vi "Configuration - Read All Module Configurations of a Specific Type.vi"(8 "error in":errorcluster, 10 "Module Type":T2=enum."Analog In Module") -> (0 "error out":errorcluster, 2 "Module Configurations":T1[](array[typedef]), 3 "Carrier Control Port":i32)   [LabVIEW 2017, in "Communications Library.lvlib"]
uses:
  Communications Library.lvlib
  Typedefs/DTACQ Device Type--Enum.ctl
  Typedefs/DTACQ Module Configuration--Cluster.ctl
  Typedefs/Functional Global Variable Action--Enum.ctl
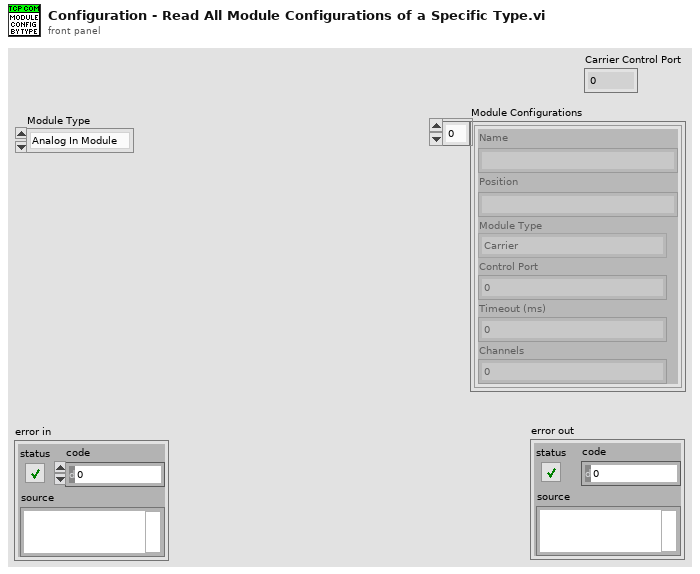
[diagram p1: front panel]
types:
  T1 = typedef "Communications Library.lvlib/DTACQ Module Configuration--Cluster.ctl" = cluster{"Name":string, "Position":string, "Module Type":T2, "Control Port":i32, "Timeout (ms)":i32, "Channels":i32}
  T2 = typedef "Communications Library.lvlib/DTACQ Device Type--Enum.ctl" = enum16{"Carrier", "Analog In Module", "Analog Out Module", "Generic Module"}
  T3 = typedef "Communications Library.lvlib/Functional Global Variable Action--Enum.ctl" = enum16{"Initialise", "Write Module Config", "Write Carrier Config", "Read"}
  T4 = typedef "Communications Library.lvlib/DTACQ Module Carrier Configuration--Cluster.ctl" = cluster{"Name":string, "IP":string, "Control Port":i32, "Timeout (ms)":i32, "Continuous Capture Port (Multiplexed)":i32, "Start HIL Shot Port":i32, "AWG Upload Port (Multiplexed)":i32, "Download Captured Data Port (Multiplexed)":i32, "Module Slots":i32, "Module Configurations":T1[]}
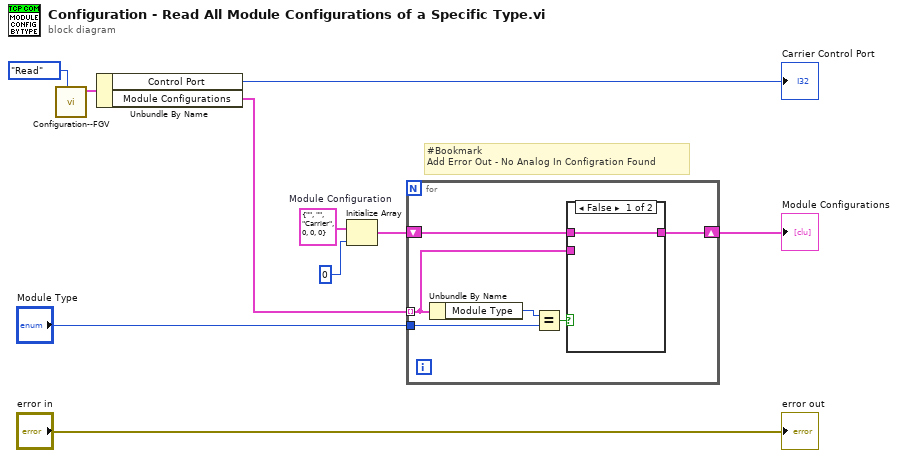
[diagram p0: block diagram]
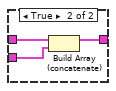
[diagram p2: hidden frame]
diagram:
  w5 = T1 {"Name"="", "Position"="", "Module Type"=enum."Carrier", "Control Port"=0, "Timeout (ms)"=0, "Channels"=0}  # Module Configuration
  # "#Bookmark\nAdd Error Out - No Analog In Configration Found"
  n1 = call "Configuration--FGV.vi"("Functional Global Action"=Functional_Global_Variable_Action--Enum."Read") -> ("Carrier Configuration Out"=w10:T4)  [unwired: 9 in, 1 out]
  n2 = Unbundle By Name(w10) -> ("Control Port"=→"Carrier Control Port":i32, "Module Configurations"=w8:T1[])
  n3 = Initialize Array(w5, 0 ("dimension size")) -> (w3:T1[])
  n4 = for {
    tunnel: w8 -> [w14] mode=indexing
    shift-right: [w13] -> w1
    shift-left: w3 -> [w16]
    tunnel: "Module Type" -> [w12]
    n5 = Unbundle By Name(w14) -> ("Module Type"=w11:T2)
    n6 = Equal?(x=w11, y=w12) -> (x = y?=w15:bool)
    n7 = case shown="False" w15 {
      tunnel: w16 -> [w17 w20]
      tunnel: w14 -> [_ w19]
      tunnel: [w17 w18] -> w13
      frame False {
      }
      frame True {
        n8 = Build Array (concatenate)(w20, w19) -> (w18:T1[])
      }
    }
  }
  "Module Configurations" <- w1
  "error out" <- "error in"
